vi "Run All.vi"(8 "Error In":errorcluster) -> (0 "Error Out":errorcluster)   [LabVIEW 2017, in "Tests.lvlib" / "Parser.lvlib"]
uses:
  Parser.lvlib
  <vilib>/addons/_JKI Toolkits/Caraya/classes/Test/Test.lvclass
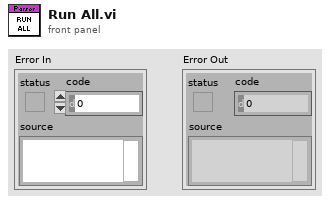
[diagram p1: front panel]
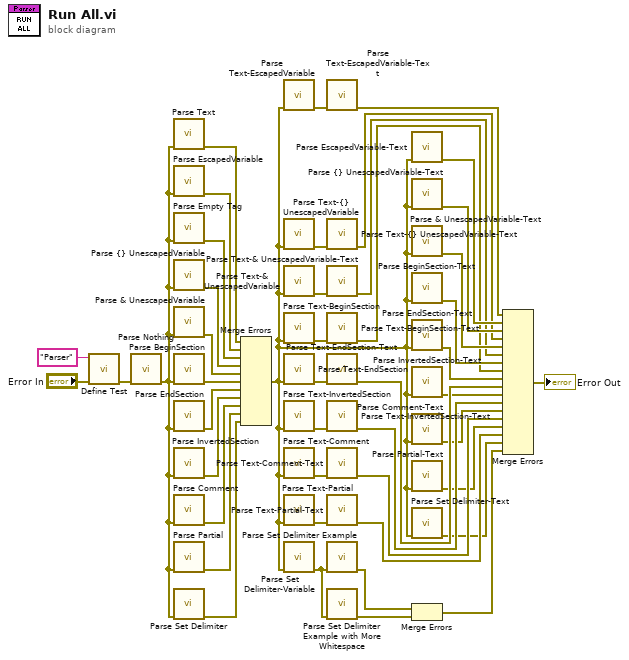
[diagram p0: block diagram]
diagram:
  n1 = call <vilib>:"Define Test.vi"("error in (no error)"="Error In", "Label (VI Title)"="Parser") -> ("error out"=w44:errorcluster)  [unwired: 9 in]
  n2 = call "Parse Nothing.vi"("Error In"=w44) -> ("Error Out"=w8:errorcluster)  [unwired: 10 in]
  n3 = call "Parse Text.vi"("Error In"=w8) -> ("Error Out"=w43:errorcluster)  [unwired: 10 in]
  n4 = call "Parse EscapedVariable.vi"("Error In"=w8) -> ("Error Out"=w42:errorcluster)  [unwired: 10 in]
  n5 = call "Parse Empty Tag.vi"("Error In"=w8) -> ("Error Out"=w37:errorcluster)  [unwired: 10 in]
  n6 = call "Parse {} UnescapedVariable.vi"("Error In"=w8) -> ("Error Out"=w36:errorcluster)  [unwired: 10 in]
  n7 = call "Parse & UnescapedVariable.vi"("Error In"=w8) -> ("Error Out"=w32:errorcluster)  [unwired: 10 in]
  n8 = call "Parse BeginSection.vi"("Error In"=w8) -> ("Error Out"=w28:errorcluster)  [unwired: 10 in]
  n9 = call "Parse EndSection.vi"("Error In"=w8) -> ("Error Out"=w23:errorcluster)  [unwired: 10 in]
  n10 = call "Parse InvertedSection.vi"("Error In"=w8) -> ("Error Out"=w19:errorcluster)  [unwired: 10 in]
  n11 = call "Parse Comment.vi"("Error In"=w8) -> ("Error Out"=w16:errorcluster)  [unwired: 10 in]
  n12 = call "Parse Partial.vi"("Error In"=w8) -> ("Error Out"=w12:errorcluster)  [unwired: 10 in]
  n13 = call "Parse Set Delimiter.vi"("Error In"=w8) -> ("Error Out"=w7:errorcluster)  [unwired: 10 in]
  n14 = Merge Errors(w43, w42, w37, w36, w32, w28, w23, w19, w16, w12, w7) -> (w5:errorcluster)
  n15 = call "Parse Text-EscapedVariable.vi"("Error In"=w5) -> ("Error Out"=w41:errorcluster)  [unwired: 10 in]
  n16 = call "Parse Text-{} UnescapedVariable.vi"("Error In"=w5) -> ("Error Out"=w33:errorcluster)  [unwired: 10 in]
  n17 = call "Parse Text-& UnescapedVariable.vi"("Error In"=w5) -> ("Error Out"=w30:errorcluster)  [unwired: 10 in]
  n18 = call "Parse Text-BeginSection.vi"("Error In"=w5) -> ("Error Out"=w25:errorcluster)  [unwired: 10 in]
  n19 = call "Parse Text-EndSection.vi"("Error In"=w5) -> ("Error Out"=w21:errorcluster)  [unwired: 10 in]
  n20 = call "Parse Text-InvertedSection.vi"("Error In"=w5) -> ("Error Out"=w17:errorcluster)  [unwired: 10 in]
  n21 = call "Parse Text-Comment.vi"("Error In"=w5) -> ("Error Out"=w13:errorcluster)  [unwired: 10 in]
  n22 = call "Parse Text-Partial.vi"("Error In"=w5) -> ("Error Out"=w9:errorcluster)  [unwired: 10 in]
  n23 = call "Parse Set Delimiter-Variable.vi"("Error In"=w5) -> ("Error Out"=w3:errorcluster)  [unwired: 10 in]
  n24 = call "Parse Text-EscapedVariable-Text.vi"("Error In"=w41) -> ("Error Out"=w40:errorcluster)  [unwired: 10 in]
  n25 = call "Parse Text-{} UnescapedVariable-Text.vi"("Error In"=w33) -> ("Error Out"=w34:errorcluster)  [unwired: 10 in]
  n26 = call "Parse Text-& UnescapedVariable-Text.vi"("Error In"=w30) -> ("Error Out"=w29:errorcluster)  [unwired: 10 in]
  n27 = call "Parse Text-BeginSection-Text.vi"("Error In"=w25) -> ("Error Out"=w26:errorcluster)  [unwired: 10 in]
  n28 = call "Parse Text-EndSection-Text.vi"("Error In"=w21) -> ("Error Out"=w22:errorcluster)  [unwired: 10 in]
  n29 = call "Parse Text-InvertedSection-Text.vi"("Error In"=w17) -> ("Error Out"=w18:errorcluster)  [unwired: 10 in]
  n30 = call "Parse Text-Comment-Text.vi"("Error In"=w13) -> ("Error Out"=w14:errorcluster)  [unwired: 10 in]
  n31 = call "Parse Text-Partial-Text.vi"("Error In"=w9) -> ("Error Out"=w10:errorcluster)  [unwired: 10 in]
  n32 = call "Parse Set Delimiter Example.vi"("Error In"=w3) -> ("Error Out"=w4:errorcluster)  [unwired: 10 in]
  n33 = call "Parse Set Delimiter Example with More Whitespace.vi"("Error In"=w3) -> ("Error Out"=w1:errorcluster)  [unwired: 10 in]
  n34 = call "Parse EscapedVariable-Text.vi"("Error In"=w5) -> ("Error Out"=w38:errorcluster)  [unwired: 10 in]
  n35 = call "Parse {} UnescapedVariable-Text.vi"("Error In"=w5) -> ("Error Out"=w35:errorcluster)  [unwired: 10 in]
  n36 = call "Parse & UnescapedVariable-Text.vi"("Error In"=w5) -> ("Error Out"=w31:errorcluster)  [unwired: 10 in]
  n37 = call "Parse BeginSection-Text.vi"("Error In"=w5) -> ("Error Out"=w27:errorcluster)  [unwired: 10 in]
  n38 = call "Parse EndSection-Text.vi"("Error In"=w5) -> ("Error Out"=w24:errorcluster)  [unwired: 10 in]
  n39 = call "Parse InvertedSection-Text.vi"("Error In"=w5) -> ("Error Out"=w20:errorcluster)  [unwired: 10 in]
  n40 = call "Parse Comment-Text.vi"("Error In"=w5) -> ("Error Out"=w15:errorcluster)  [unwired: 10 in]
  n41 = call "Parse Partial-Text.vi"("Error In"=w5) -> ("Error Out"=w11:errorcluster)  [unwired: 10 in]
  n42 = call "Parse Set Delimiter-Text.vi"("Error In"=w5) -> ("Error Out"=w6:errorcluster)  [unwired: 10 in]
  n43 = Merge Errors(w4, w1) -> (w2:errorcluster)
  n44 = Merge Errors(w40, w38, w35, w34, w31, w29, w27, w26, w24, w22, w20, w18, w15, w14, w11, w10, w6, w2) -> (→"Error Out":errorcluster)
